vi "ClimbExecute.vi"(8 "error in (no error)":errorcluster) -> (0 "error out":errorcluster)   [LabVIEW 2023]
uses:
  <vilib>/Rock Robotics/WPI/ThirdParty/JAS_Junk/TrajLib/VI/BoolCmd_Recv_Internal.vi
  <vilib>/Rock Robotics/WPI/ThirdParty/JAS_Junk/TrajLib/Timer_New.vi
  <vilib>/Rock Robotics/WPI/ThirdParty/JAS_Junk/TrajLib/VI/BoolCmd_ObtainQueue.vi
  <vilib>/Rock Robotics/Network Tables/NT Write Number.vi
  <vilib>/Rock Robotics/Network Tables/NT Write Boolean.vi
  <vilib>/Utility/semaphor.llb/Obtain Semaphore Reference.vi
  <vilib>/Rock Robotics/WPI/ThirdParty/JAS_Junk/TrajLib/Timer_Reset.vi
  <vilib>/Rock Robotics/WPI/ThirdParty/JAS_Junk/TrajLib/Timer_Start.vi
  <vilib>/Rock Robotics/WPI/ThirdParty/JAS_Junk/TrajLib/Timer_Stop.vi
  <vilib>/Rock Robotics/WPI/ThirdParty/JAS_Junk/TrajLib/Timer_HasPeriodPassedOnce.vi
  <vilib>/Rock Robotics/WPI/ThirdParty/JAS_Junk/TrajLib/Trajectory_Library.lvlib
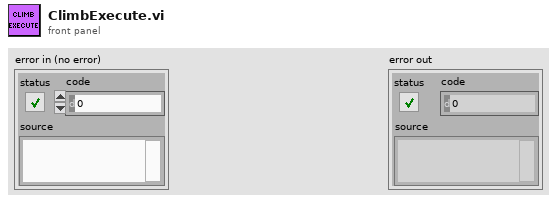
[diagram p1: front panel]
types:
  T1 = typedef "WPI_MotorControlDeviceRef.ctl" = cluster{"DeviceStatus":errorcluster, "Type":T2, "PWM":cluster{"PWM Channel":T3, "DeadBand":T4}, "CAN":cluster{"Device Number":u8, "SetOutput VI Ref":variant, "GetOutput VI Ref":variant, "Enable VI Ref":variant, "Disable VI Ref":variant, "Data":variant}, "Invert":bool, "DIO PWM":cluster{"PWM \"Enable\" Channel":T3, "DIOChannel":T5, "PWM Rate":dbl}}
  T2 = typedef "WPI_MotorControlType.ctl" = enum16{"PWM", "CAN", "DIO PWM"}
  T3 = typedef "FPGA_DIOPWMChannel.ctl" = enum8{"PWM 0", "PWM 1", "PWM 2", "PWM 3", "PWM 4", "PWM 5", "PWM 6", "PWM 7", "PWM 8", "PWM 9", "PWM MXP 0", "PWM MXP 1", "PWM MXP 2", "PWM MXP 3", "PWM MXP 4", "PWM MXP 5", "PWM MXP 6", "PWM MXP 7", "PWM MXP 8", "PWM MXP 9", "Invalid"}
  T4 = typedef "WPI_PWMDeadband.ctl" = cluster{"Name":string, "maxPositivePwm":i32, "minPositivePwm":i32, "centerPwm":i32, "maxNegativePwm":i32, "minNegativePwm":i32, "angularRange":u16}
  T5 = typedef "FPGA_DIOChannel.ctl" = enum8{"DIO 0", "DIO 1", "DIO 2", "DIO 3", "DIO 4", "DIO 5", "DIO 6", "DIO 7", "DIO 8", "DIO 9", "DIO MXP 0", "DIO MXP 1", "DIO MXP 2", "DIO MXP 3", "DIO MXP 4", "DIO MXP 5", "DIO MXP 6", "DIO MXP 7", "DIO MXP 8", "DIO MXP 9", "DIO MXP 10", "DIO MXP 11", "DIO MXP 12", "DIO MXP 13", "DIO MXP 14", "DIO MXP 15", "SPI Port CS1", "SPI Port CS2", "SPI Port CS3", "SPI Port MISO", "SPI Port MOSI", "Invalid"}
  T6 = typedef "Trajectory_Library.lvlib/PosCtrl_Tuning_Type.ctl" = cluster{"Slope":dbl, "Offset":dbl, "Error Deadband":dbl, "At Reference Count":i32, "Negate Output":bool, "Max Allowd Position":dbl, "Min Allowd Position":dbl}
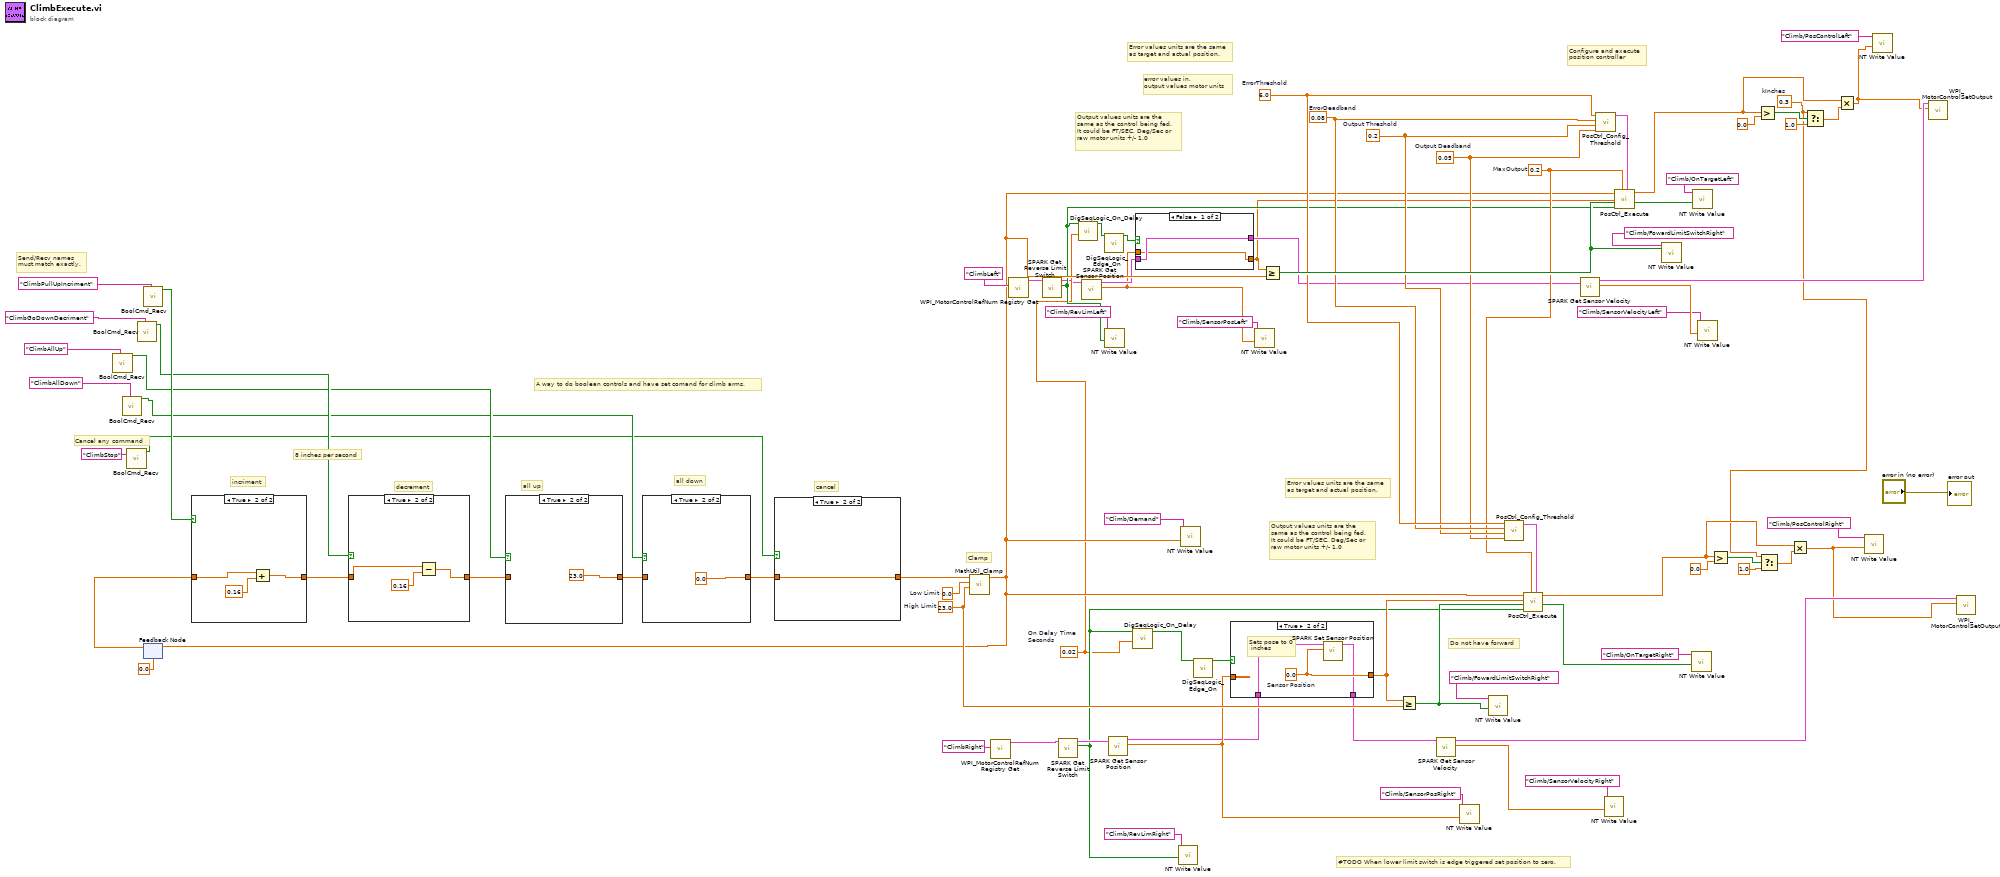
[diagram p0: block diagram]
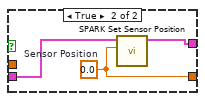
[diagram p2: hidden frame]
diagram:
  w3 = 0.3  # kInches
  w22 = 0.02  # On Delay Time Seconds
  w41 = 23.0  # High Limit
  w50 = 0.0  # Low Limit
  w29 = 0.2  # MaxOutput
  w33 = 6.0  # ErrorThreshold
  w32 = 0.08  # ErrorDeadband
  w31 = 0.2  # Output Threshold
  w30 = 0.05  # Output Deadband
  # "#TODO When lower limit switch is edge triggered set position to zero."
  # "cancel"
  # "Clamp"
  # "8 inches per second"
  # "all down"
  # "all up"
  # "decrement"
  # "incriment"
  # "Cancel any command"
  # "Send/Recv names\nmust match exactly."
  # "A way to do boolean controls and have set comand for climb arms."
  # "error values in.\noutput values motor units"
  # "Do not have forward"
  # "Output values units are the\nsame as the control being fed.  \nIt could be FT/SEC, Deg/Sec or\nraw motor units +/- 1.0"
  # "Error values units are the same \nas target and actual position."
  # "Output values units are the\nsame as the control being fed.  \nIt could be FT/SEC, Deg/Sec or\nraw motor units +/- 1.0"
  # "Error values units are the same \nas target and actual position."
  # "Configure and execute \nposition controller"
  n1 = call <vilib>:"BoolCmd_Recv.vi"("Command Name"="ClimbAllUp") -> ("New Request"=w45:bool)  [unwired: 9 in, 1 out]
  n2 = call <vilib>:"BoolCmd_Recv.vi"("Command Name"="ClimbAllDown") -> ("New Request"=w44:bool)  [unwired: 9 in, 1 out]
  n3 = call <vilib>:"BoolCmd_Recv.vi"("Command Name"="ClimbStop") -> ("New Request"=w43:bool)  [unwired: 9 in, 1 out]
  n4 = call <vilib>:"BoolCmd_Recv.vi"("Command Name"="ClimbGoDownDecriment") -> ("New Request"=w46:bool)  [unwired: 9 in, 1 out]
  n5 = call <vilib>:"BoolCmd_Recv.vi"("Command Name"="ClimbPullUpIncriment") -> ("New Request"=w47:bool)  [unwired: 9 in, 1 out]
  n6 = feedback #1(0.0 ("false")) -> (w54:dbl)
  n7 = case shown="True" w47 {
    tunnel: w54 -> [w84 w87]
    tunnel: [w84 w85] -> w53
    frame False {
    }
    frame True {
      n8 = Add(x=w87, y=0.16) -> (x+y=w85:dbl)
    }
  }
  n9 = case shown="True" w46 {
    tunnel: w53 -> [w88 w90]
    tunnel: [w88 w89] -> w52
    frame False {
    }
    frame True {
      n10 = Subtract(x=w90, y=0.16) -> (x-y=w89:dbl)
    }
  }
  n11 = case shown="True" w45 {
    tunnel: w52 -> [w92 _]
    tunnel: [w92 23.0 ("y")] -> w51
    frame False {
    }
    frame True {
    }
  }
  n12 = case shown="True" w44 {
    tunnel: w51 -> [w94 _]
    tunnel: [w94 0.0 ("y")] -> w49
    frame False {
    }
    frame True {
    }
  }
  n13 = case shown="True" w43 {
    tunnel: w49 -> [w96 w97]
    tunnel: [w96 w97] -> w48
    frame False {
    }
    frame True {
    }
  }
  n14 = call <vilib>:"MathUtil_Clamp.vi"("High Limit"=w41, "Low Limit"=w50, "Value"=w48) -> ("Result"=w24:dbl)  [unwired: 8 in]
  n15 = feedback-in #1(w24) -> ()
  n16 = call <vilib>:"WPI_MotorControlRefNum Registry Get.vi"("refnum name"="ClimbRight") -> ("MotorControlDevRef"=w76:T1)  [unwired: 9 in, 1 out]
  n17 = call <vilib>:"WPI_MotorControlRefNum Registry Get.vi"("refnum name"="ClimbLeft") -> ("MotorControlDevRef"=w82:T1)  [unwired: 9 in, 1 out]
  n18 = call <vilib>:"SPARK Get Reverse Limit Switch.vi"("MotorControlDevRef in"=w82) -> ("Hard Limit Rev"=w23:bool, "MotorControlDevRef out"=w19:T1)  [unwired: 7 in, 2 out]
  n19 = call <vilib>:"SPARK Get Reverse Limit Switch.vi"("MotorControlDevRef in"=w76) -> ("Hard Limit Rev"=w27:bool, "MotorControlDevRef out"=w74:T1)  [unwired: 7 in, 2 out]
  n20 = call <vilib>:"DigSeqLogic_On_Delay.vi"("Delay"=w22, "Input"=w23) -> ("Output"=w21:bool)  [unwired: 8 in, 1 out]
  n21 = call <vilib>:"SPARK Get Sensor Position.vi"("MotorControlDevRef in"=w19) -> ("Sensor Position"=w16:dbl, "MotorControlDevRef out"=w18:T1)  [unwired: 7 in, 2 out]
  n22 = call <vilib>:"DigSeqLogic_Edge_On.vi"("Input"=w21) -> ("On Edge"=w20:bool)  [unwired: 10 in]
  n23 = call-poly <vilib>:"NT Write Value.vi"("value"=w23, "name"="Climb/RevLimLeft") -> ()  [unwired: 9 in, 1 out]
  n24 = call <vilib>:"SPARK Get Sensor Position.vi"("MotorControlDevRef in"=w74) -> ("Sensor Position"=w35:dbl, "MotorControlDevRef out"=w26:T1)  [unwired: 7 in, 2 out]
  n25 = call <vilib>:"DigSeqLogic_On_Delay.vi"("Delay"=w22, "Input"=w27) -> ("Output"=w36:bool)  [unwired: 8 in, 1 out]
  n26 = case shown="False" w20 {
    tunnel: w18 -> [w99 w102]
    tunnel: [w99 w101] -> w17
    tunnel: w16 -> [w98 _]
    tunnel: [w98 w100] -> w15
    frame False {
    }
    frame True {
      w100 = 0.0  # Sensor Position
      n27 = call <vilib>:"SPARK Set Sensor Position.vi"("Position"=w100, "MotorControlDeviceRef"=w102) -> ("MotorControlDeviceRef"=w101:T1)  [unwired: 8 in, 1 out]
    }
  }
  n28 = call-poly <vilib>:"NT Write Value.vi"("value"=w27, "name"="Climb/RevLimRight") -> ()  [unwired: 9 in, 1 out]
  n29 = call-poly <vilib>:"NT Write Value.vi"("value"=w24, "name"="Climb/Demand") -> ()  [unwired: 9 in, 1 out]
  n30 = call <vilib>:"DigSeqLogic_Edge_On.vi"("Input"=w36) -> ("On Edge"=w28:bool)  [unwired: 10 in]
  n31 = case shown="True" w28 {
    tunnel: w35 -> [w104 _]
    tunnel: [w104 w107] -> w34
    tunnel: w26 -> [w103 w106]
    tunnel: [w103 w105] -> w25
    frame False {
    }
    frame True {
      w107 = 0.0  # Sensor Position
      # "Sets pose to 0\n inches"
      n32 = call <vilib>:"SPARK Set Sensor Position.vi"("Position"=w107, "MotorControlDeviceRef"=w106) -> ("MotorControlDeviceRef"=w105:T1)  [unwired: 8 in, 1 out]
    }
  }
  n33 = call-poly <vilib>:"NT Write Value.vi"("value"=w16, "name"="Climb/SensorPosLeft") -> ()  [unwired: 9 in, 1 out]
  n34 = Greater Or Equal?(x=w15, y=w24) -> (x >= y?=w37:bool)
  n35 = Greater Or Equal?(x=w34, y=w41) -> (x >= y?=w39:bool)
  n36 = call <vilib>:"SPARK Get Sensor Velocity.vi"("MotorControlDevRef in"=w25) -> ("Sensor Velocity"=w71:dbl, "MotorControlDevRef out"=w61:T1)  [unwired: 7 in, 2 out]
  n37 = call-poly <vilib>:"NT Write Value.vi"("value"=w35, "name"="Climb/SensorPosRight") -> ()  [unwired: 9 in, 1 out]
  n38 = call-poly <vilib>:"NT Write Value.vi"("value"=w39, "name"="Climb/FowardLimitSwitchRight") -> ()  [unwired: 9 in, 1 out]
  n39 = call <vilib>:"PosCtrl_Config_Threshold.vi"("Output Deadband"=w30, "Output Threshold"=w31, "ErrorDeadband"=w32, "ErrorThreshold"=w33) -> ("PosCtrl_Config_Params"=w64:T6)  [unwired: 7 in]
  n40 = call <vilib>:"PosCtrl_Execute.vi"("PosCtrl_Config_Params"=w64, "MaxOutput"=w29, "Rev Limit Switch"=w27, "Fwd Limit Switch"=w39, "CurrentPosition"=w34, "TargetPosition"=w24) -> ("OnTarget"=w63:bool, "Output"=w4:dbl)  [unwired: 3 in, 1 out]
  n41 = call <vilib>:"SPARK Get Sensor Velocity.vi"("MotorControlDevRef in"=w17) -> ("Sensor Velocity"=w78:dbl, "MotorControlDevRef out"=w69:T1)  [unwired: 7 in, 2 out]
  n42 = call <vilib>:"PosCtrl_Config_Threshold.vi"("Output Deadband"=w30, "Output Threshold"=w31, "ErrorDeadband"=w32, "ErrorThreshold"=w33) -> ("PosCtrl_Config_Params"=w83:T6)  [unwired: 7 in]
  n43 = call-poly <vilib>:"NT Write Value.vi"("value"=w71, "name"="Climb/SensorVelocityRight") -> ()  [unwired: 9 in, 1 out]
  n44 = call <vilib>:"PosCtrl_Execute.vi"("PosCtrl_Config_Params"=w83, "MaxOutput"=w29, "Rev Limit Switch"=w23, "Fwd Limit Switch"=w37, "CurrentPosition"=w15, "TargetPosition"=w24) -> ("OnTarget"=w66:bool, "Output"=w10:dbl)  [unwired: 3 in, 1 out]
  n45 = call-poly <vilib>:"NT Write Value.vi"("value"=w37, "name"="Climb/FowardLimitSwitchRight") -> ()  [unwired: 9 in, 1 out]
  n46 = call-poly <vilib>:"NT Write Value.vi"("value"=w63, "name"="Climb/OnTargetRight") -> ()  [unwired: 9 in, 1 out]
  n47 = call-poly <vilib>:"NT Write Value.vi"("value"=w66, "name"="Climb/OnTargetLeft") -> ()  [unwired: 9 in, 1 out]
  n48 = call-poly <vilib>:"NT Write Value.vi"("value"=w78, "name"="Climb/SensorVelocityLeft") -> ()  [unwired: 9 in, 1 out]
  n49 = Greater?(x=w4, y=0.0) -> (0:w8:bool)
  n50 = Greater?(x=w10, y=0.0) -> (0:w13:bool)
  n51 = Select(t=w3, s=w8, f=1.0) -> (s? t:f=w6:dbl)
  n52 = Multiply(x=w4, y=w6) -> (x*y=w2:dbl)
  n53 = Select(t=w3, s=w13, f=1.0) -> (s? t:f=w11:dbl)
  n54 = Multiply(x=w10, y=w11) -> (x*y=w1:dbl)
  n55 = call-poly <vilib>:"NT Write Value.vi"("value"=w2, "name"="Climb/PosControlRight") -> ()  [unwired: 9 in, 1 out]
  n56 = call-poly <vilib>:"NT Write Value.vi"("value"=w1, "name"="Climb/PosControlLeft") -> ()  [unwired: 9 in, 1 out]
  n57 = call <vilib>:"WPI_MotorControlSetOutput.vi"("Output"=w1, "MotorControlDevRef"=w69) -> ()  [unwired: 7 in, 3 out]
  n58 = call <vilib>:"WPI_MotorControlSetOutput.vi"("Output"=w2, "MotorControlDevRef"=w61) -> ()  [unwired: 7 in, 3 out]
  "error out" <- "error in (no error)"
